vi "Query Multi Eval Meas Trigger Source Catalog.vi"(8 "error in (no error)":errorcluster, 10 "Instance (1)":T1=1, 11 "VISA resource name":refnum<visa-resource-name>) -> (0 "error out":errorcluster, 2 "Trigger Source Catalog":string[](array[string]), 3 "VISA resource name out":refnum<visa-resource-name>)   [LabVIEW 2020, in "Rohde&Schwarz CMWXP NR FR1 Measurement.lvlib"]
doc: "Lists all trigger source values that can be set using TRIGger:NRSub:MEAS<i>:MEValuation:SOURce.\n\nAttribute:\nRSCMWXPNRFR1M_ATTR_MULTI_EVAL_MEAS_TRIGGER_SOURCE_CATALOG\n\nRemote-control command:\nTRIGger:NRSub:MEAS<i>:MEValuation:CATalog:SOURce?"
uses:
  <instrlib>/Rohde&Schwarz CMWXP NR FR1 Measurement/Rohde&Schwarz CMWXP NR FR1 Measurement.lvlib
  <instrlib>/Rohde&Schwarz CMWXP NR FR1 Measurement/Private/_Instance.ctl
  <instrlib>/Rohde&Schwarz CMWXP NR FR1 Measurement/Private/rsidr_core.llb/rsidr_core.lvlib
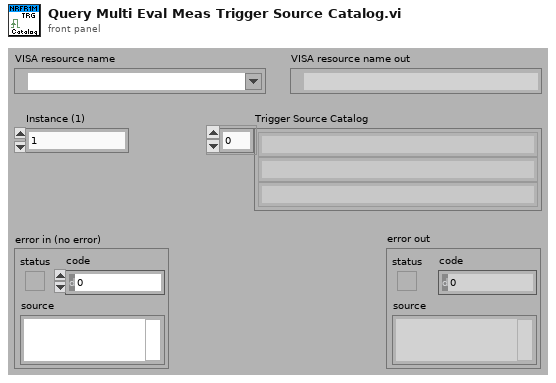
[diagram p1: front panel]
types:
  T1 = typedef "Rohde&Schwarz CMWXP NR FR1 Measurement.lvlib/_Instance.ctl" = i32
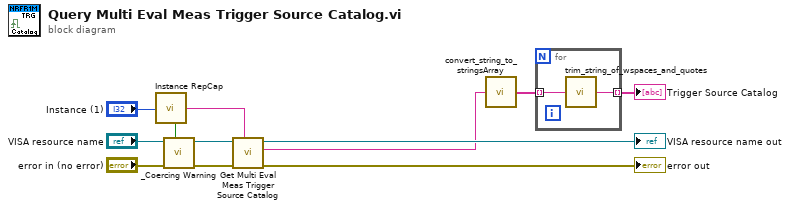
[diagram p0: block diagram]
diagram:
  n1 = call <instrlib>:"Instance RepCap.vi"("Instance In"="Instance (1)") -> ("In Range?"=w1:bool, "RepCap Identifier Out"=w9:string)  [unwired: 1 in]
  n2 = call <instrlib>:"_Coercing Warning.vi"("In Range?"=w1, "error in (no error)"="error in (no error)", "VISA resource name"="VISA resource name") -> ("error out"=w3:errorcluster, "VISA resource name out"=w2:refnum<visa-resource-name>)  [unwired: 7 in]
  n3 = call "Get Multi Eval Meas Trigger Source Catalog"("Repeated Capabilities"=w9, "error in (no error)"=w3, "instrument handle"=w2) -> ("error out"=→"error out":errorcluster, "Multi Eval Meas Trigger Source Catalog"=w8:string, "instrument handle out"=→"VISA resource name out":refnum<visa-resource-name>)  [unwired: 6 in]
  n4 = call <instrlib>:"convert_string_to_stringsArray.vi"("String in"=w8) -> ("string array out"=w7:string[])  [unwired: 3 in, 1 out]
  n5 = for {
    tunnel: w7 -> [w14] mode=indexing
    tunnel: [w13] -> w6 mode=indexing
    n6 = call <instrlib>:"trim_string_of_wspaces_and_quotes.vi"("String in"=w14) -> ("String out"=w13:string)  [unwired: 4 in]
  }
  "Trigger Source Catalog" <- w6
